vi "Waveform Editor UI.vi"() -> ()   [LabVIEW 2020]
uses:
  Libraries/Waveform Obj Class/Waveform Gen/Controls/repeat scale.ctl
  Libraries/Waveform Obj Class/Square Wave/Controls/Slope Type.ctl
  Libraries/Waveform Obj Class/Waveform Gen/Waveform Gen.lvclass
  Libraries/Waveform Obj Class/Square Wave/Square Wave.lvclass
panel:
  out "Graph":dbl[](graph)
  in  "Mem_Start 2":bool
  in  "Mem_Start":bool
  in  "WF Gen_Wait":u8(ring) caption="Wait" items=["0us", "166us", "332us", "498us", "664us", "830us", "996us", "1162us", "1328us", "1494us", "1660us", "1826us", "1992us", "2158us", "2324us", "2490us"]
  in  "Mem Update":bool
  in  "RTP Stop":bool
  in  "RTP Start":bool
  in  "WF Gen_Voltage Range":dbl(ring) caption="VD_Clamp" items=["0.00V"=0.0, "0.04V"=0.04, "0.08V"=0.08, "0.12V"=0.12, "0.16V"=0.16, "0.20V"=0.2, "0.24V"=0.24, "0.28V"=0.28, "0.32V"=0.32, "0.36V"=0.36, "0.40V"=0.4, "0.44V"=0.44, "0.48V"=0.48, "0.52V"=0.52, "0.56V"=0.56, "0.60V"=0.6, "0.64V"=0.64, "0.68V"=0.68, "0.72V"=0.72, "0.76V"=0.76, "0.80V"=0.8, "0.84V"=0.84, "0.88V"=0.88, "0.92V"=0.92, "0.96V"=0.96, "1.00V"=1.0, "1.04V"=1.04, "1.08V"=1.08, "1.12V"=1.12, "1.16V"=1.16, "1.20V"=1.2, "1.24V"=1.24, "1.28V"=1.28, "1.32V"=1.32, "1.36V"=1.36, "1.40V"=1.4, "1.44V"=1.44, "1.48V"=1.48, "1.52V"=1.52, "1.56V"=1.56, "1.60V"=1.6, "1.64V"=1.64, "1.68V"=1.68, "1.72V"=1.72, "1.76V"=1.76, "1.80V"=1.8, "1.84V"=1.84, "1.88V"=1.88, "1.92V"=1.92, "1.96V"=1.96, "2.00V"=2.0, "2.04V"=2.04, "2.08V"=2.08, "2.12V"=2.12, "2.16V"=2.16, "2.20V"=2.2, "2.24V"=2.24, "2.28V"=2.28, "2.32V"=2.32, "2.36V"=2.36, "2.40V"=2.4, "2.44V"=2.44, "2.48V"=2.48, "2.52V"=2.52, "2.56V"=2.56, "2.60V"=2.6, "2.64V"=2.64, "2.68V"=2.68, "2.72V"=2.72, "2.76V"=2.76, "2.80V"=2.8, "2.84V"=2.84, "2.88V"=2.88, "2.92V"=2.92, "2.96V"=2.96, "3.00V"=3.0, "3.04V"=3.04, "3.08V"=3.08, "3.12V"=3.12, "3.16V"=3.16, "3.20V"=3.2, "3.24V"=3.24, "3.28V"=3.28, "3.32V"=3.32, "3.36V"=3.36, "3.40V"=3.4, "3.44V"=3.44, "3.48V"=3.48, "3.52V"=3.52, "3.56V"=3.56, "3.60V"=3.6, "3.64V"=3.64, "3.68V"=3.68, "3.72V"=3.72, "3.76V"=3.76, "3.80V"=3.8, "3.84V"=3.84, "3.88V"=3.88, "3.92V"=3.92, "3.96V"=3.96, "4.00V"=4.0, "4.04V"=4.04, "4.08V"=4.08, "4.12V"=4.12, "4.16V"=4.16, "4.20V"=4.2, "4.24V"=4.24, "4.28V"=4.28, "4.32V"=4.32, "4.36V"=4.36, "4.40V"=4.4, "4.44V"=4.44, "4.48V"=4.48, "4.52V"=4.52, "4.56V"=4.56, "4.60V"=4.6, "4.64V"=4.64, "4.68V"=4.68, "4.72V"=4.72, "4.76V"=4.76, "4.80V"=4.8, "4.84V"=4.84, "4.88V"=4.88, "4.92V"=4.92, "4.96V"=4.96, "5.00V"=5.0, "5.04V"=5.04, "5.08V"=5.08, "5.12V"=5.12, "5.16V"=5.16, "5.20V"=5.2, "5.24V"=5.24, "5.28V"=5.28, "5.32V"=5.32, "5.36V"=5.36, "5.40V"=5.4, "5.44V"=5.44, "5.48V"=5.48, "5.52V"=5.52, "5.56V"=5.56, "5.60V"=5.6, "5.64V"=5.64, "5.68V"=5.68, "5.72V"=5.72, "5.76V"=5.76, "5.80V"=5.8, "5.84V"=5.84, "5.88V"=5.88, "5.92V"=5.92, "5.96V"=5.96, "6.00V"=6.0, "6.04V"=6.04, "6.08V"=6.08, "6.12V"=6.12, "6.16V"=6.16, "6.20V"=6.2, "6.24V"=6.24, "6.28V"=6.28, "6.32V"=6.32, "6.36V"=6.36, "6.40V"=6.4, "6.44V"=6.44, "6.48V"=6.48, "6.52V"=6.52, "6.56V"=6.56, "6.60V"=6.6, "6.64V"=6.64, "6.68V"=6.68, "6.72V"=6.72, "6.76V"=6.76, "6.80V"=6.8, "6.84V"=6.84, "6.88V"=6.88, "6.92V"=6.92, "6.96V"=6.96, "7.00V"=7.0, "7.04V"=7.04, "7.08V"=7.08, "7.12V"=7.12, "7.16V"=7.16, "7.20V"=7.2, "7.24V"=7.24, "7.28V"=7.28, "7.32V"=7.32, "7.36V"=7.36, "7.40V"=7.4, "7.44V"=7.44, "7.48V"=7.48, "7.52V"=7.52, "7.56V"=7.56, "7.60V"=7.6, "7.64V"=7.64, "7.68V"=7.68, "7.72V"=7.72, "7.76V"=7.76, "7.80V"=7.8, "7.84V"=7.84, "7.88V"=7.88, "7.92V"=7.92, "7.96V"=7.96, "8.00V"=8.0, "8.04V"=8.04, "8.08V"=8.08, "8.12V"=8.12, "8.16V"=8.16, "8.20V"=8.2, "8.24V"=8.24, "8.28V"=8.28, "8.32V"=8.32, "8.36V"=8.36, "8.40V"=8.4, "8.44V"=8.44, "8.48V"=8.48, "8.52V"=8.52, "8.56V"=8.56, "8.60V"=8.6, "8.64V"=8.64, "8.68V"=8.68, "8.72V"=8.72, "8.76V"=8.76, "8.80V"=8.8, "8.84V"=8.84, "8.88V"=8.88, "8.92V"=8.92, "8.96V"=8.96, "9.00V"=9.0, "9.04V"=9.04, "9.08V"=9.08, "9.12V"=9.12, "9.16V"=9.16, "9.20V"=9.2, "9.24V"=9.24, "9.28V"=9.28, "9.32V"=9.32, "9.36V"=9.36, "9.40V"=9.4, "9.44V"=9.44, "9.48V"=9.48, "9.52V"=9.52, "9.56V"=9.56, "9.60V"=9.6, "9.64V"=9.64, "9.68V"=9.68, "9.72V"=9.72, "9.76V"=9.76, "9.80V"=9.8, "9.84V"=9.84, "9.88V"=9.88, "9.92V"=9.92, "9.96V"=9.96, "10.00V"=10.0, "10.04V"=10.04, "10.08V"=10.08, "10.12V"=10.12, "10.16V"=10.16, "10.20V"=10.2]
  in  "Import":bool
  out "WF List_Total Bytes":i32 caption="Total :" format="%d Byte"
  out "WF Seq_Total Bytes":i32 caption="Total :" format="%d Byte"
  in  "Export":bool
  in  "WF List_Load File":bool
  in  "WF List_Save File":bool
  in  "WF List_Delete":bool
  in  "WF List_Rename":bool
  in  "WF List_Down":bool
  in  "WF List_Up":bool
  in  "WF Seq_Modify":bool
  in  "WF Seq_Add to List":bool
  in  "WF Seq_Delete":bool
  in  "WF Seq_Rename":bool
  in  "WF Seq_Down":bool
  in  "WF Seq_Up":bool
  in  "WF Seq_View":bool
  in  "WF Gen_Modify":bool
  in  "WF Gen_Add to Seq":bool
  in  "WF Gen_Setting":T3={"Waveform Type"=0, "Freq."=160.0, "Scale"=1.0, "Cycle"=1.0, "Repeat Type"=enum."Normal", "Square_Slope Length"=25, "Square_Slope"=enum."Exp."} {"Scale" min=-1.0 max=1.0; "Waveform Type" items=["Sine", "Square", "Triangle", "Sawtooth", "Auto Track", "Auto Brake (Square)", "Auto Brake (Sine)"]}
  in  "WF Gen_Sampling Rate":u32(ring)=8000 caption="PWM" items=["24kHz"=24000, "48kHz"=48000, "96kHz"=96000, "12kHz"=12000]
  in  "WF Seq":i32[](listbox)
  in  "WF List":i32[](listbox)
  # "Waveform Editor"
  # "Waveform Setting"
  # "Waveform Generate"
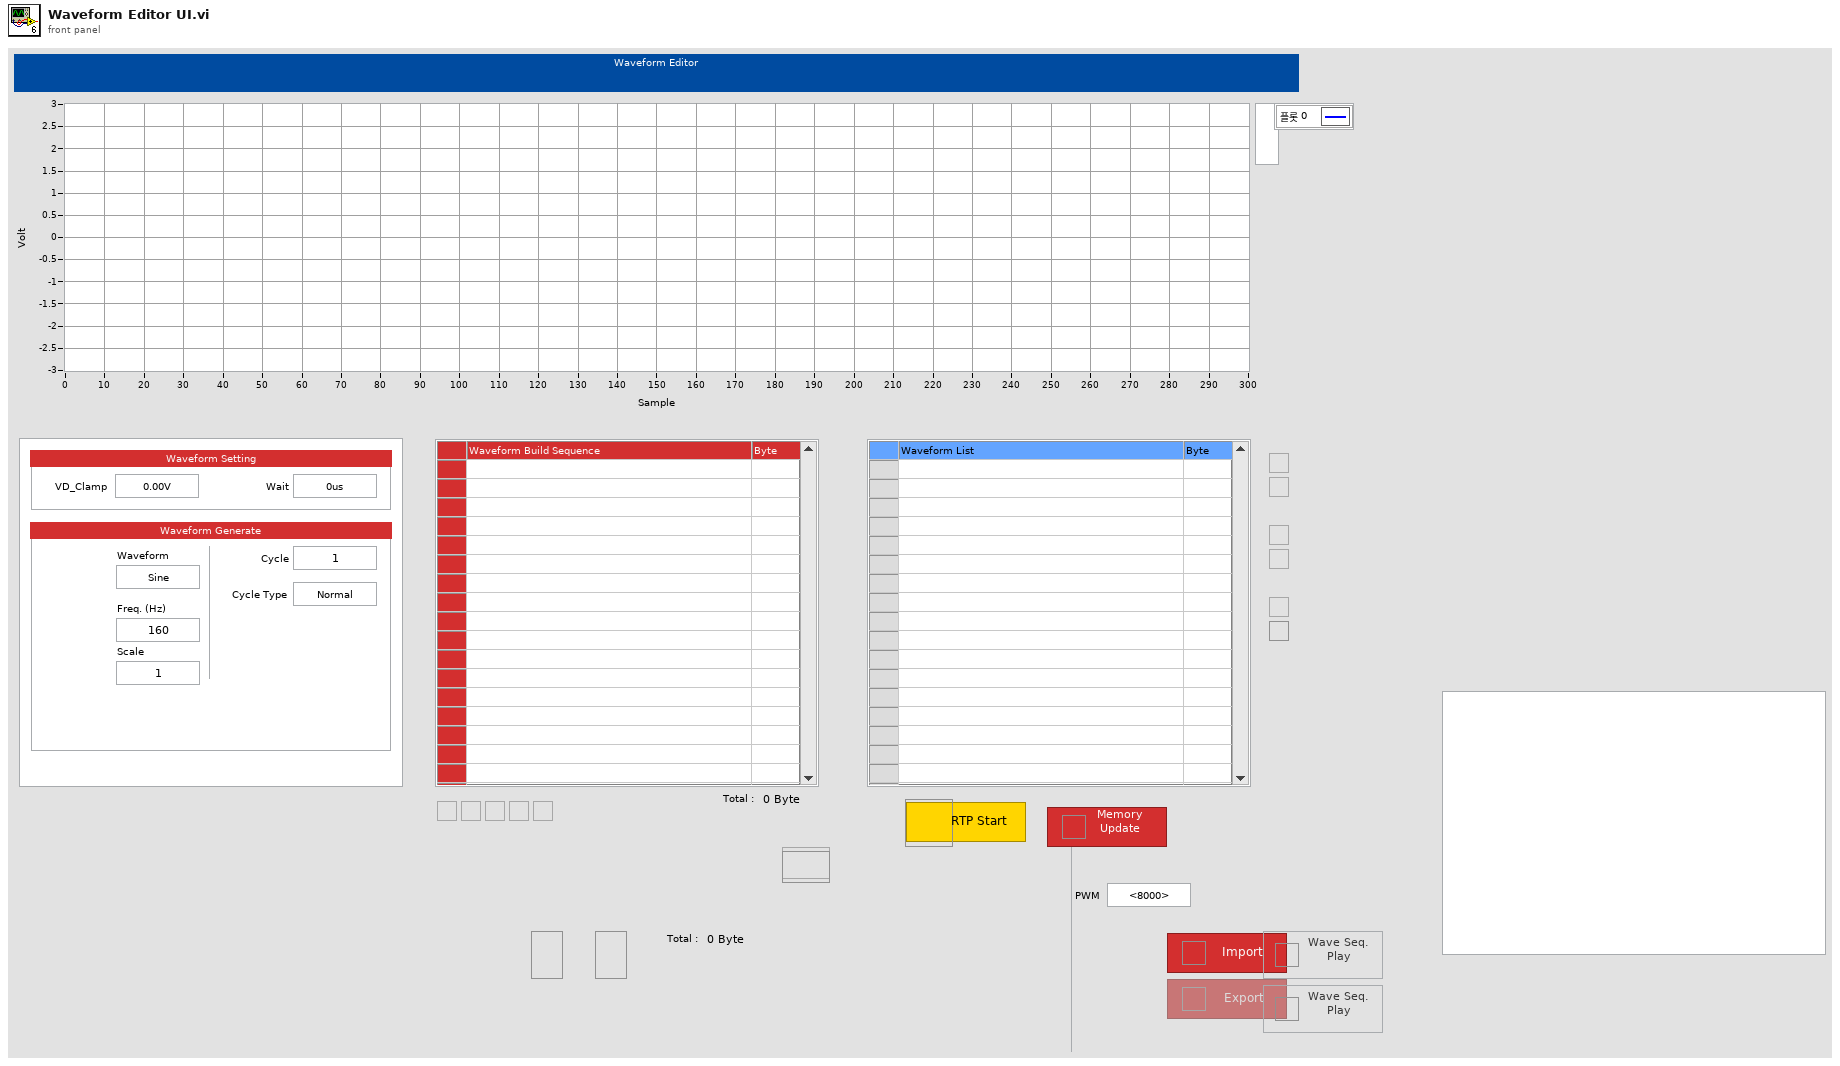
[diagram p1: front panel]
types:
  T1 = typedef "Waveform Gen.lvclass/repeat scale.ctl" = enum16{"Normal", "Lin. Up", "Lin. Down", "Exp. Up", "Exp. Down"}
  T2 = typedef "Square Wave.lvclass/Slope Type.ctl" = enum16{"None", "Lin.", "Exp."}
  T3 = cluster{"Waveform Type":u16, "Freq.":dbl, "Scale":dbl, "Cycle":dbl, "Repeat Type":T1, "Square_Slope Length":u32, "Square_Slope":T2}
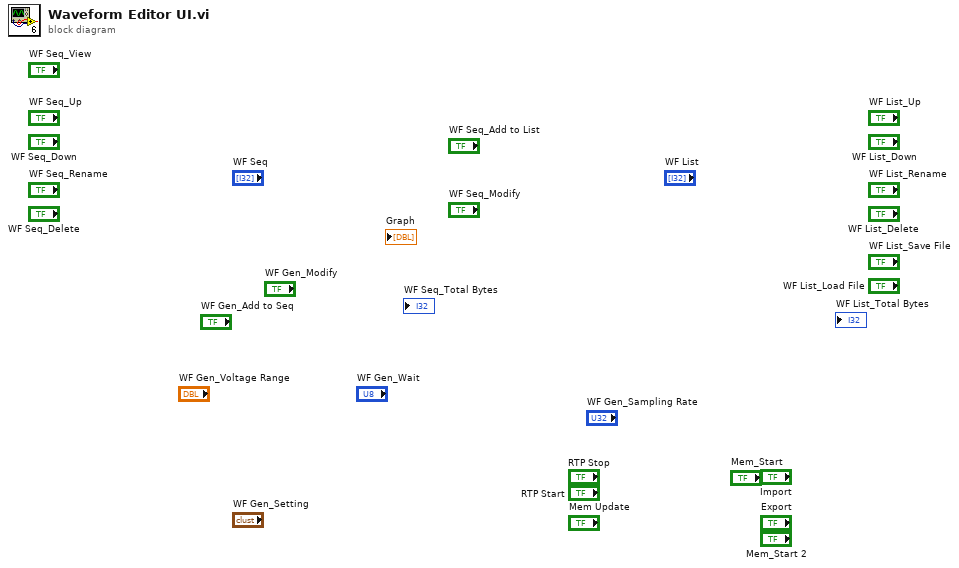
[diagram p0: block diagram]
diagram:
